vi "Convert.vi"() -> ()   [LabVIEW 2014]
panel:
  in  "Path":path
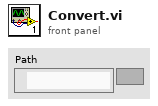
[diagram p1: front panel]
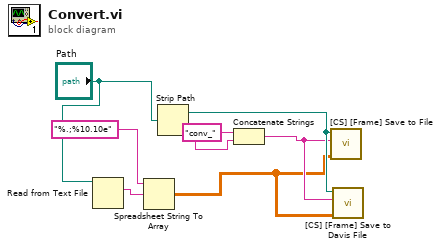
[diagram p0: block diagram]
diagram:
  n1 = Read from Text File(file (use dialog)="Path") -> (text=w3:string)  [unwired: 3 in, 3 out]
  n2 = Spreadsheet String To Array(format string="%.;%10.10e" ("format (%.3f)"), spreadsheet string=w3) -> (array=w4:dbl[][])  [unwired: 2 in]
  n3 = Strip Path(path="Path") -> (stripped path=w6:path, name=w7:string)
  n4 = Concatenate Strings("conv_" ("string"), w7) -> (w5:string)
  n5 = call "[CS] [Frame] Save to File.vi"("array"=w4, "Name"=w5, "base path"=w6) -> ()  [unwired: 9 in]
  n6 = call "[CS] [Frame] Save to Davis File.vi"("array"=w4, "Name"=w5, "base path"=w6) -> ()  [unwired: 9 in]
